vi "Get_Cluster_Argument0.vi"(1 "Clust Refnum":refnum<vi>, 2 "Argument List In":string[](array[string])) -> (0 "Argument List Out":string[](array[string]))   [LabVIEW 2011]
doc: "This VI parses an argument to find it's text value. For example, given an argument in the form of Arg(\"some text\"), it would return \"some text\", without quotation marks."
uses:
  high_level_proc/source_dilution.ctl
  high_level_proc/source_noDilution.ctl
panel:
  out "error out":errorcluster
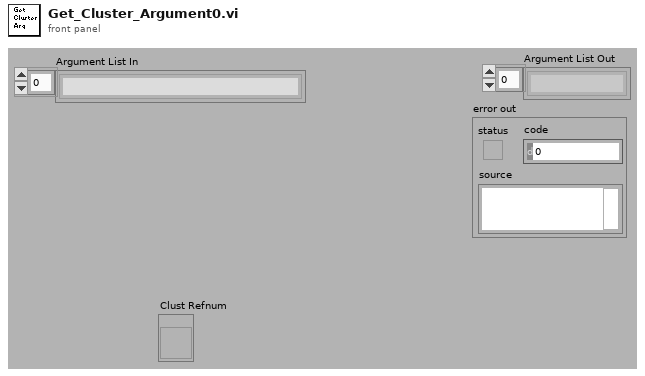
[diagram p1: front panel]
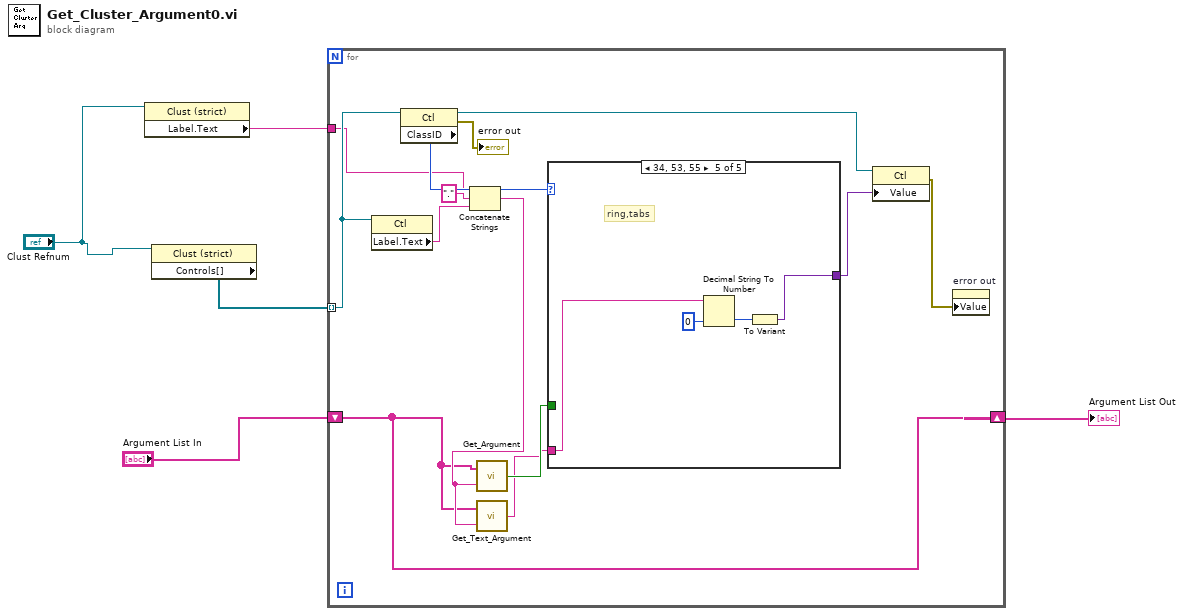
[diagram p0: block diagram]
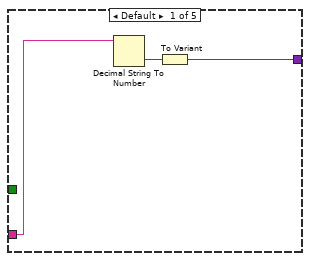
[diagram p2: hidden frame]
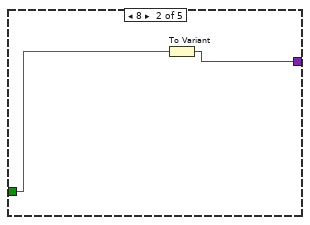
[diagram p3: hidden frame]
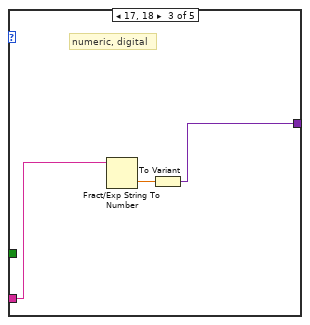
[diagram p4: hidden frame]
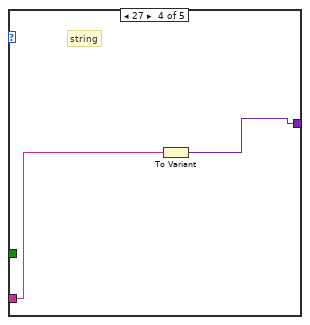
[diagram p5: hidden frame]
diagram:
  n1 = property class="Clust (strict)"(reference="Clust Refnum") -> ("Label.Text"=w1:string)  [unwired: 1 in, 2 out]
  n2 = property class="Clust (strict)"(reference="Clust Refnum") -> ("Controls[]"=w3:refnum<vi>[])  [unwired: 1 in, 2 out]
  n3 = for {
    tunnel: w3 -> [w18] mode=indexing
    shift-right: [w9] -> w4
    shift-left: "Argument List In" -> [w9]
    tunnel: w1 -> [w13]
    n4 = property class="Ctl"(reference=w18) -> ("Label.Text"=w15:string)  [unwired: 1 in, 2 out]
    n5 = property class="Ctl"(reference=w18) -> (reference out=w6:refnum<vi>, error out=→"error out":errorcluster, "ClassID"=w17:u32)  [unwired: 1 in]
    n6 = Concatenate Strings(w13, "." ("string"), w15) -> (w12:string)
    n7 = call "Get_Argument.vi"("Argument"=w12, "Argument List"=w9) -> ("Enabled"=w11:bool)
    n8 = call "Get_Text_Argument.vi"("Argument"=w12, "Argument List"=w9) -> ("Text"=w10:string)
    n9 = case shown="34, 53, 55" w17 {
      tunnel: w11 -> [_ w23 _ _ _]
      tunnel: w10 -> [w19 _ w26 w28 w30]
      tunnel: [w20 w22 w24 w27 w29] -> w7
      frame Default {
        n10 = Decimal String To Number(string=w19) -> (number=w21:i32)  [unwired: 2 in, 1 out]
        n11 = To Variant(anything=w21) -> (Variant=w20:variant)
      }
      frame 8 {
        n12 = To Variant(anything=w23) -> (Variant=w22:variant)
      }
      frame 17, 18 {
        # "numeric, digital"
        n13 = Fract/Exp String To Number(string=w26) -> (number=w25:dbl)  [unwired: 3 in, 1 out]
        n14 = To Variant(anything=w25) -> (Variant=w24:variant)
      }
      frame 27 {
        # "string"
        n15 = To Variant(anything=w28) -> (Variant=w27:variant)
      }
      frame 34, 53, 55 {
        # "ring,tabs"
        n16 = Decimal String To Number(string=w30, default (0L)=u16 0 ("default (0 I32)")) -> (number=w32:u16)  [unwired: 1 in, 1 out]
        n17 = To Variant(anything=w32) -> (Variant=w29:variant)
      }
    }
    n18 = property class="Ctl"(reference=w6, "Value"=w7) -> (error out=w8:errorcluster)  [unwired: 1 in, 1 out]
    n19 = property on="error out" class="Clust (strict)"("Value"=w8) -> ()  [unwired: 2 in, 2 out]
  }
  "Argument List Out" <- w4
